vi "Init State Data.vi"(4 "load data":T1={"max address"=0.0, "memory"="Digital Pattern Gen Memory 0"}, 6 "settings.<user name>":T3, 11 "state data in":T2) -> (3 "state data out":T2)   [LabVIEW 2015, in "Engine Simulation Toolkit.lvlib" / "Digital Pattern Generation.lvlib"]
uses:
  Digital Pattern Generation.lvlib
  Settings.ctl
  state data.ctl
  Load Data.ctl
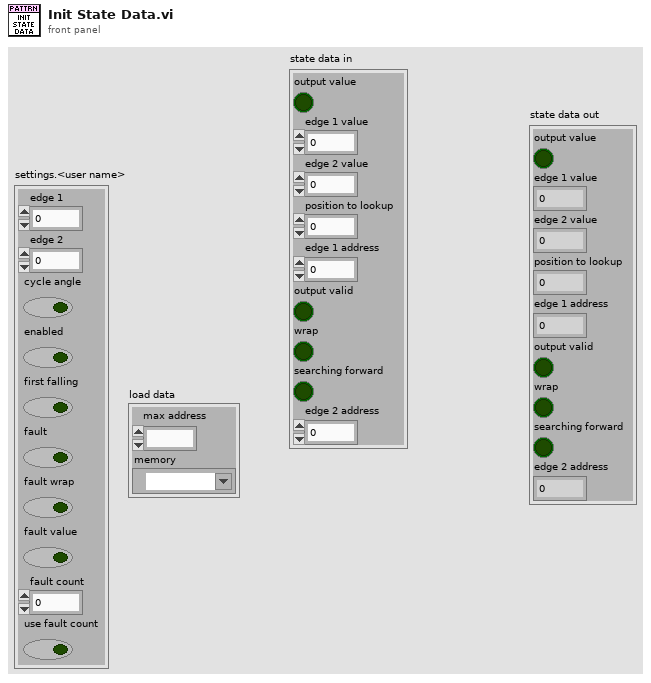
[diagram p1: front panel]
types:
  T1 = typedef "Engine Simulation Toolkit.lvlib/Digital Pattern Generation.lvlib/Load Data.ctl" = cluster{"max address":fxp<+,11,11>, "memory":refnum<k21>}
  T2 = typedef "Engine Simulation Toolkit.lvlib/Digital Pattern Generation.lvlib/state data.ctl" = cluster{"output value":bool, "edge 1 value":u16, "edge 2 value":u16, "position to lookup":u16, "edge 1 address":fxp<+,11,11>, "output valid":bool, "wrap":bool, "searching forward":bool, "edge 2 address":fxp<+,11,11>}
  T3 = typedef "Engine Simulation Toolkit.lvlib/Digital Pattern Generation.lvlib/Settings.ctl" = cluster{"edge 1":u16, "edge 2":u16, "cycle angle":bool, "enabled":bool, "first falling":bool, "fault":bool, "fault wrap":bool, "fault value":bool, "fault count":fxp<+,4,4>, "use fault count":bool}
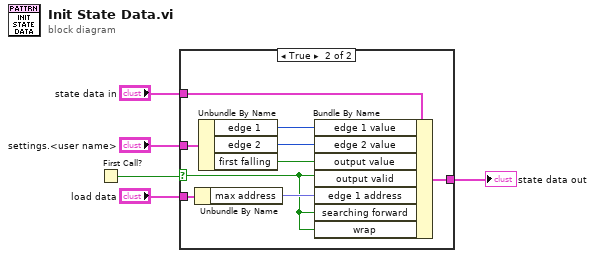
[diagram p0: block diagram]
diagram:
  n1 = First Call?() -> (First Call?: T/F=w5:bool)
  n2 = case shown="True" w5 {
    selector: w5 -> [_ w8]
    tunnel: "settings.<user name>" -> [_ w14]
    tunnel: [w6 w11] -> w3
    tunnel: "state data in" -> [w6 w15]
    tunnel: "load data" -> [_ w10]
    frame False {
    }
    frame True {
      n3 = Unbundle By Name(w10) -> ("max address"=w9:fxp<+,11,11>)
      n4 = Unbundle By Name(w14) -> ("edge 1"=w13:u16, "edge 2"=w12:u16, "first falling"=w7:bool)
      n5 = Bundle By Name(cluster=w15, "edge 1 value"=w13, "edge 2 value"=w12, "output value"=w7, "output valid"=w8, "edge 1 address"=w9, "searching forward"=w8, "wrap"=w8) -> (w11:T2)
    }
  }
  "state data out" <- w3
